vi "Destory for traverse.vi"(8 "error in (no error)":errorcluster caption="错误输入（无错误）", 11 "Class in":refnum<class "PanelRootNode.lvclass"> caption="DNL_LabVIEW Object in") -> (0 "error out":errorcluster caption="错误输出", 3 "Class out":refnum<class "PanelRootNode.lvclass"> caption="DNL_LabVIEW Object out")   [LabVIEW 2016, in "PanelRootNode.lvclass"]
uses:
  PanelRootNode.lvclass
  C:/Users/CL/Desktop/ZcDAQprj0811/ZcDAQprj/Modules/DAQ-Display/PanelSplitToolkit/PanelLinkNode/PanelLinkNode.lvclass
  PanelObject/PanelObject.lvclass
  PanelLinkNode/PanelLinkNode.lvclass/PanelLinkNode.ctl
  PanelLinkNode/PanelLinkNode.lvclass
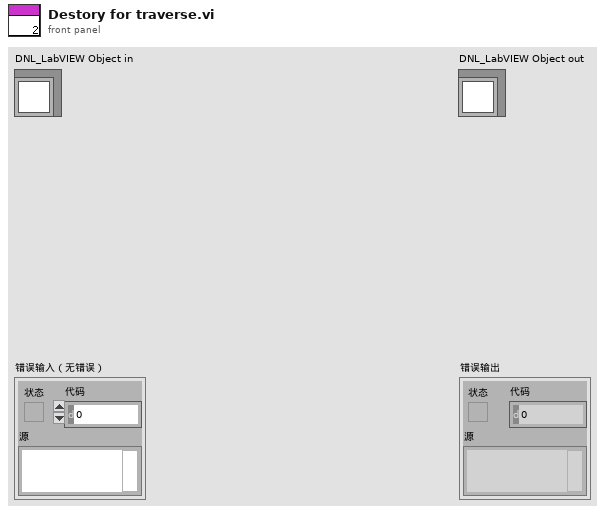
[diagram p1: front panel]
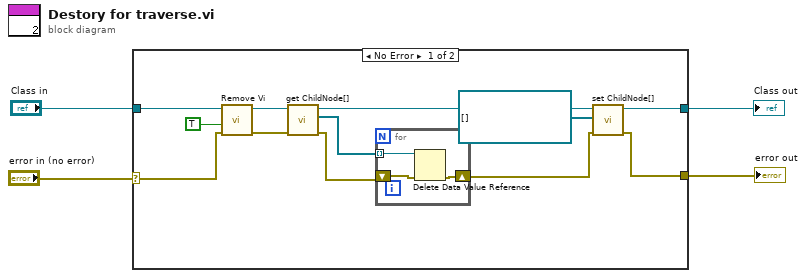
[diagram p0: block diagram]
diagram:
  n1 = case shown="No Error" "error in (no error)" {
    selector: "error in (no error)" -> [w7 w21]
    tunnel: [w5 w21] -> w3
    tunnel: [w9 w20] -> w1
    tunnel: "Class in" -> [w15 w20]
    frame No Error {
      n2 = call-dynamic "Remove Vi.vi"("error in"=w7, "Abort VI"=TRUE, "PanelDataNode 输入"=w15) -> ("error out"=w13:errorcluster, "PanelDataNode 输出"=w14:refnum<class "PanelRootNode.lvclass">)  [unwired: 5 in, 2 out]
      n3 = call "get ChildNode[].vi"("error in (no error)"=w13, "PanelLinkNode输入"=w14) -> ("error out"=w11:errorcluster, "ChildNode*[]"=w12:refnum<data-value>[], "PanelLinkNode输出"=w10:refnum<class "PanelRootNode.lvclass">)  [unwired: 7 in]
      n4 = for {
        tunnel: w12 -> [w19] mode=indexing
        shift-right: [w17] -> w6
        shift-left: w11 -> [w18]
        n5 = Delete Data Value Reference(data value reference=w19, error in=w18) -> (error out=w17:errorcluster)  [unwired: 1 out]
      }
      n6 = call "set ChildNode[].vi"("error in (no error)"=w6, "ChildNode*[]"=refnum<data-value>[] [], "PanelLinkNode输入"=w10) -> ("error out"=w5:errorcluster, "PanelLinkNode输出"=w9:refnum<class "PanelRootNode.lvclass">)  [unwired: 7 in]
    }
    frame Error {
    }
  }
  "error out" <- w3
  "Class out" <- w1
